vi "Create Frame Host LLP Packets.vi"(0 "frame configuration":T1={"pixel data type"=enum."RAW 8", "horizontal resolution"=0, "vertical resolution"=0, "virtual channel"=0.0, "include line sync packets"=FALSE}, 5 "frame number":u16, 11 "error in (no error)":errorcluster) -> (4 "frame packets":T3[](array[typedef]), 15 "error out":errorcluster)   [LabVIEW 2023, in "GettingStarted_Gen_148X_Host.lvlib"]
uses:
  GettingStarted_Gen_148X_Host.lvlib
  <instrlib>/FlexRIO/CSI-2/v2/Host/Types/Host LLP Packet.ctl
  <instrlib>/FlexRIO/CSI-2/v2/FPGA/Types/LLP Packet Header.ctl
  <instrlib>/FlexRIO/CSI-2/v2/FPGA/Types/LLP Packet Footer.ctl
  Types/Frame Data Configuration.ctl
  <instrlib>/FlexRIO/CSI-2/v2/Common/Types/LLP Data Type.ctl
  <instrlib>/FlexRIO/CSI-2/v2/FPGA/NI CSI-2 API FPGA v2.lvlib
  <instrlib>/FlexRIO/CSI-2/v2/Host/NI CSI-2 API Host v2.lvlib
  <instrlib>/FlexRIO/CSI-2/v2/Common/NI CSI-2 API Common v2.lvlib
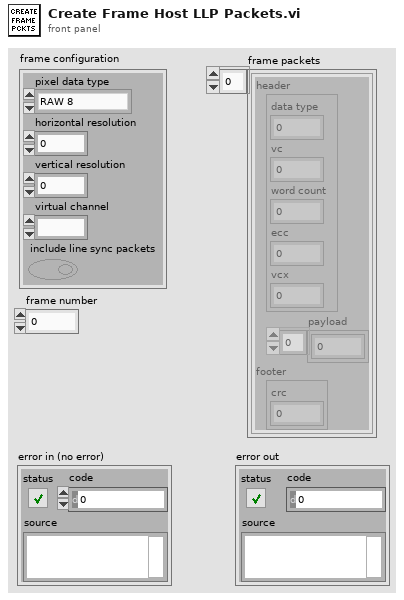
[diagram p1: front panel]
types:
  T1 = typedef "GettingStarted_Gen_148X_Host.lvlib/Frame Data Configuration.ctl" = cluster{"pixel data type":T2, "horizontal resolution":u16, "vertical resolution":u16, "virtual channel":fxp<+,4,4>, "include line sync packets":bool}
  T2 = typedef "NI CSI-2 API Common v2.lvlib/LLP Data Type.ctl" = enum8{"Frame Start", "Frame End", "Line Start", "Line End", "End of Transmission", "Reserved 0", "Reserved 1", "Reserved 2", "Generic Short Packet 1", "Generic Short Packet 2", "Generic Short Packet 3", "Generic Short Packet 4", "Generic Short Packet 5", "Generic Short Packet 6", "Generic Short Packet 7", "Generic Short Packet 8", "Null", "Blanking Data", "Embedded 8-bit non Image Data", "Generic Long Packet 1", "Generic Long Packet 2", "Generic Long Packet 3", "Generic Long Packet 4", "Reserved 3", "YUV420 8-bit", "YUV420 10-bit", "Legacy YUV420 8-bit", "Reserved 4", "YUV420 8-bit Chroma Shifted", "YUV420 10-bit Chroma Shifted", "YUV422 8-bit", "YUV422 10-bit", "RGB444", "RGB555", "RGB565", "RGB666", "RGB888", "Reserved 5", "Reserved 6", "RAW 24", "RAW 6", "RAW 7", "RAW 8", "RAW 10", "RAW 12", "RAW 14", "RAW 16", "RAW 20", "User Defined 8-bit Data 1", "User Defined 8-bit Data 2", "User Defined 8-bit Data 3", "User Defined 8-bit Data 4", "User Defined 8-bit Data 5", "User Defined 8-bit Data 6", "User Defined 8-bit Data 7", "User Defined 8-bit Data 8", "USL Command", "Reserved 7", "Reserved 8", "Reserved 9", "Reserved 10", "Reserved 11", "Reserved 12", "LRTE EPD Spacer"}
  T3 = typedef "NI CSI-2 API Host v2.lvlib/Host LLP Packet.ctl" = cluster{"header":T4, "payload":u8[], "footer":T5}
  T4 = typedef "NI CSI-2 API FPGA v2.lvlib/LLP Packet Header.ctl" = cluster{"word count":u16, "ecc":fxp<+,6,6>, "vcx":fxp<+,2,2>, "data type":fxp<+,6,6>, "vc":fxp<+,2,2>}
  T5 = typedef "NI CSI-2 API FPGA v2.lvlib/LLP Packet Footer.ctl" = cluster{"crc":u16}
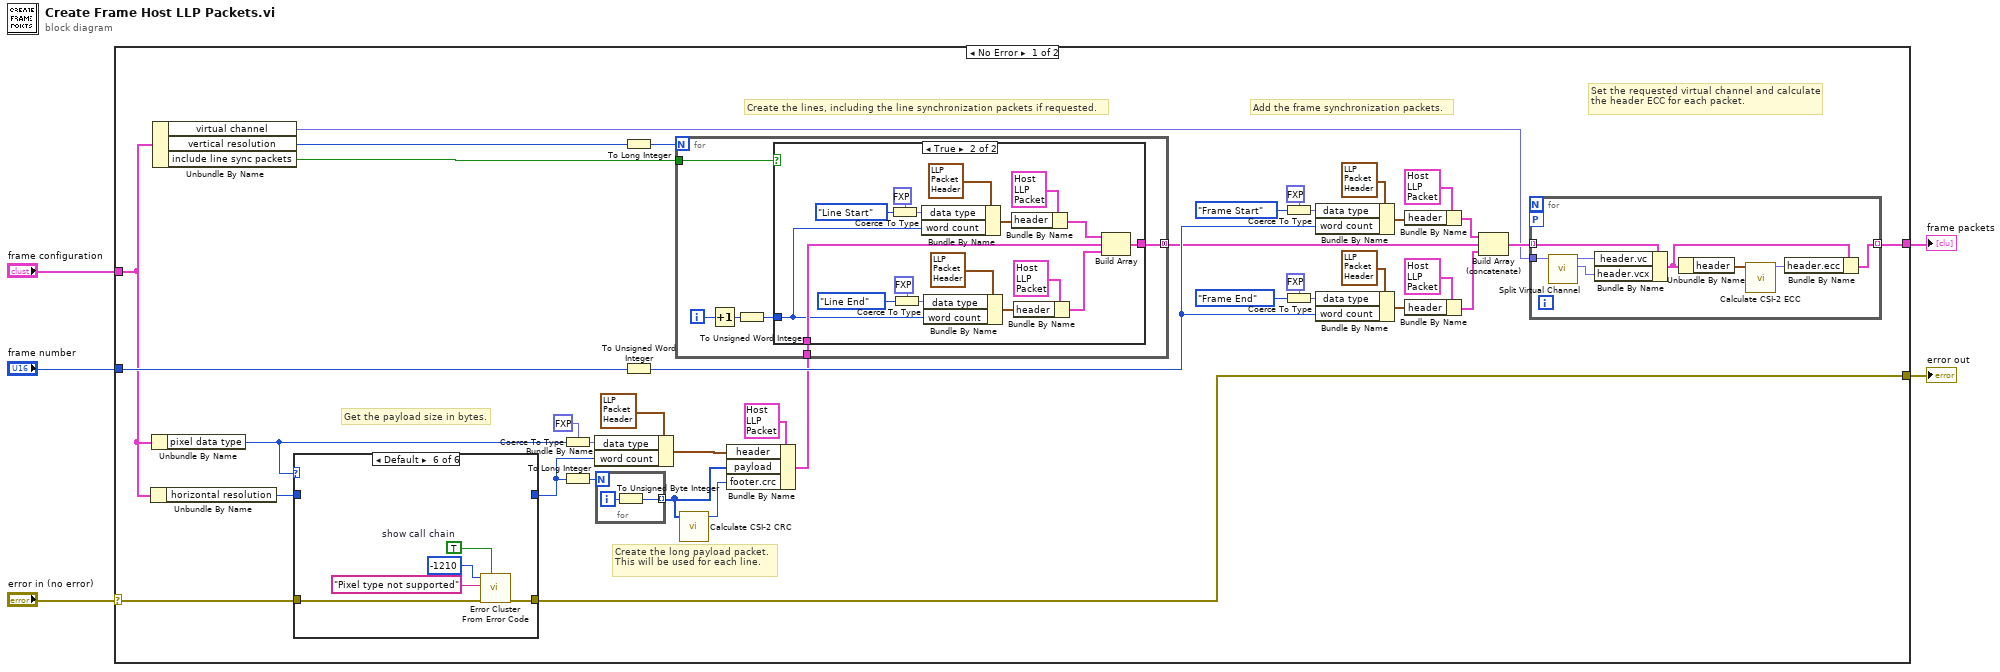
[diagram p0: block diagram]
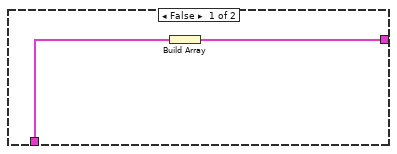
[diagram p2: hidden frame]
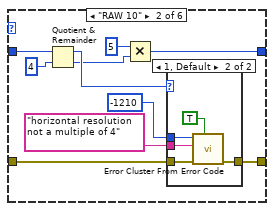
[diagram p4: hidden frame]
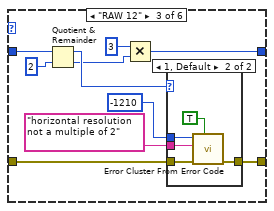
[diagram p6: hidden frame]
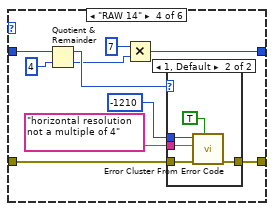
[diagram p8: hidden frame]
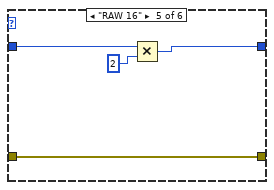
[diagram p10: hidden frame]
diagram:
  n1 = case shown="No Error" "error in (no error)" {
    selector: "error in (no error)" -> [w8 w138]
    tunnel: [w32 _] -> w5
    tunnel: [w43 w138] -> w3
    tunnel: "frame number" -> [w14 _]
    tunnel: "frame configuration" -> [w9 _]
    frame No Error {
      # "Set the requested virtual channel and calculate the header ECC for each packet."
      # "Add the frame synchronization packets."
      # "Create the lines, including the line synchronization packets if requested."
      # "Create the long payload packet.  This will be used for each line."
      # "Get the payload size in bytes."
      n2 = Unbundle By Name(w9) -> ("horizontal resolution"=w12:u16)
      n3 = Unbundle By Name(w9) -> ("pixel data type"=w13:T2)
      n4 = Unbundle By Name(w9) -> ("virtual channel"=w10:fxp<+,4,4>, "vertical resolution"=w11:u16, "include line sync packets"=w7:bool)
      n5 = case shown="Default" w13 {
        tunnel: w12 -> [w78 w81 w97 w113 w130 _]
        tunnel: [w78 w80 w96 w112 w128 _] -> w37
        tunnel: w8 -> [w77 w88 w104 w120 w127 w134]
        tunnel: [w77 w85 w101 w117 w127 w133] -> w43
        frame "RAW 8" {
        }
        frame "RAW 10" {
          n6 = Quotient & Remainder(x=w81, y=u16 4) -> (x-y*floor(x/y)=w83:u16, floor(x/y)=w79:u16)
          n7 = Multiply(x=u16 5 ("y"), y=w79) -> (x*y=w80:u16)
          n8 = case shown="1, Default" w83 {
            tunnel: w88 -> [w89 w91]
            tunnel: -1210 ("code") -> [_ w93]
            tunnel: "horizontal resolution not a multiple of 4" ("source") -> [_ w92]
            tunnel: [w89 w90] -> w85
            frame 0 {
            }
            frame 1, Default {
              n9 = call <vilib>:"Error Cluster From Error Code.vi"("show call chain? (False)"=TRUE ("show call chain"), "error in (no error)"=w91, "error message (\"\")"=w92, "error code (0)"=w93) -> ("error out"=w90:errorcluster)  [unwired: 5 in]
            }
          }
        }
        frame "RAW 12" {
          n10 = Quotient & Remainder(x=w97, y=u16 2) -> (x-y*floor(x/y)=w99:u16, floor(x/y)=w95:u16)
          n11 = Multiply(x=u16 3 ("y"), y=w95) -> (x*y=w96:u16)
          n12 = case shown="1, Default" w99 {
            tunnel: w104 -> [w105 w107]
            tunnel: -1210 ("code") -> [_ w109]
            tunnel: "horizontal resolution not a multiple of 2" ("source") -> [_ w108]
            tunnel: [w105 w106] -> w101
            frame 0 {
            }
            frame 1, Default {
              n13 = call <vilib>:"Error Cluster From Error Code.vi"("show call chain? (False)"=TRUE ("show call chain"), "error in (no error)"=w107, "error message (\"\")"=w108, "error code (0)"=w109) -> ("error out"=w106:errorcluster)  [unwired: 5 in]
            }
          }
        }
        frame "RAW 14" {
          n14 = Quotient & Remainder(x=w113, y=u16 4) -> (x-y*floor(x/y)=w115:u16, floor(x/y)=w111:u16)
          n15 = Multiply(x=u16 7 ("y"), y=w111) -> (x*y=w112:u16)
          n16 = case shown="1, Default" w115 {
            tunnel: w120 -> [w121 w123]
            tunnel: -1210 ("code") -> [_ w125]
            tunnel: "horizontal resolution not a multiple of 4" ("source") -> [_ w124]
            tunnel: [w121 w122] -> w117
            frame 0 {
            }
            frame 1, Default {
              n17 = call <vilib>:"Error Cluster From Error Code.vi"("show call chain? (False)"=TRUE ("show call chain"), "error in (no error)"=w123, "error message (\"\")"=w124, "error code (0)"=w125) -> ("error out"=w122:errorcluster)  [unwired: 5 in]
            }
          }
        }
        frame "RAW 16" {
          n18 = Multiply(x=w130, y=u16 2) -> (x*y=w128:u16)
        }
        frame Default {
          w135 = TRUE  # show call chain
          n19 = call <vilib>:"Error Cluster From Error Code.vi"("show call chain? (False)"=w135, "error in (no error)"=w134, "error message (\"\")"="Pixel type not supported" ("source"), "error code (0)"=-1210 ("code")) -> ("error out"=w133:errorcluster)  [unwired: 5 in]
        }
      }
      n20 = Coerce To Type(0:w13, 1:fxp<+,6,6> 0.0 ("data type")) -> (2:w40:fxp<+,6,6>)
      n21 = To Long Integer(number=w37) -> (32bit integer=w42:i32)
      n22 = Bundle By Name(cluster=T4 {"word count"=0, "ecc"=0.0, "vcx"=0.0, "data type"=0.0, "vc"=0.0} ("header"), "data type"=w40, "word count"=w37) -> (w41:T4)
      n23 = for {
        N: w42 -> [_]
        tunnel: [w136] -> w36 mode=indexing
        i -> [w137]
        n24 = To Unsigned Byte Integer(number=w137) -> (unsigned 8bit integer=w136:u8)
      }
      n25 = To Long Integer(number=w11) -> (32bit integer=w15:i32)
      n26 = To Unsigned Word Integer(number=w14) -> (unsigned 16bit integer=w19:u16)
      n27 = call <instrlib>:"Calculate CSI-2 CRC.vi"("payload"=w36) -> ("crc"=w35:u16)  [unwired: 10 in]
      n28 = Bundle By Name(cluster=T3 {"header"={"word count"=0, "ecc"=0.0, "vcx"=0.0, "data type"=0.0, "vc"=0.0}, "payload"=[], "footer"={"crc"=0}}, "header"=w41, "payload"=w36, "footer.crc"=w35) -> (w6:T3)
      n29 = for {
        N: w15 -> [_]
        tunnel: w7 -> [w45]
        tunnel: w6 -> [w46]
        tunnel: [w44] -> w18 mode=concatenating
        i -> [w47]
        n30 = Increment(x=w47) -> (x+1=w49:i32)
        n31 = To Unsigned Word Integer(number=w49) -> (unsigned 16bit integer=w48:u16)
        n32 = case shown="True" w45 {
          tunnel: w48 -> [_ w53]
          tunnel: w46 -> [w51 w55]
          tunnel: [w50 w52] -> w44
          frame False {
            n33 = Build Array(w51) -> (w50:T3[])
          }
          frame True {
            n34 = Coerce To Type(0:LLP_Data_Type."Line Start" ("Enum"), 1:fxp<+,6,6> 0.0 ("data type")) -> (2:w64:fxp<+,6,6>)
            n35 = Coerce To Type(0:LLP_Data_Type."Line End" ("Enum"), 1:fxp<+,6,6> 0.0 ("data type")) -> (2:w58:fxp<+,6,6>)
            n36 = Bundle By Name(cluster=T4 {"word count"=0, "ecc"=0.0, "vcx"=0.0, "data type"=0.0, "vc"=0.0} ("header"), "data type"=w64, "word count"=w53) -> (w67:T4)
            n37 = Bundle By Name(cluster=T4 {"word count"=0, "ecc"=0.0, "vcx"=0.0, "data type"=0.0, "vc"=0.0} ("header"), "data type"=w58, "word count"=w53) -> (w61:T4)
            n38 = Bundle By Name(cluster=T3 {"header"={"word count"=0, "ecc"=0.0, "vcx"=0.0, "data type"=0.0, "vc"=0.0}, "payload"=[], "footer"={"crc"=0}}, "header"=w67) -> (w56:T3)
            n39 = Bundle By Name(cluster=T3 {"header"={"word count"=0, "ecc"=0.0, "vcx"=0.0, "data type"=0.0, "vc"=0.0}, "payload"=[], "footer"={"crc"=0}}, "header"=w61) -> (w54:T3)
            n40 = Build Array(w56, w55, w54) -> (w52:T3[])
          }
        }
      }
      n41 = Coerce To Type(0:LLP_Data_Type."Frame Start" ("Enum"), 1:fxp<+,6,6> 0.0 ("data type")) -> (2:w25:fxp<+,6,6>)
      n42 = Coerce To Type(0:LLP_Data_Type."Frame End" ("Enum"), 1:fxp<+,6,6> 0.0 ("data type")) -> (2:w26:fxp<+,6,6>)
      n43 = Bundle By Name(cluster=T4 {"word count"=0, "ecc"=0.0, "vcx"=0.0, "data type"=0.0, "vc"=0.0} ("header"), "data type"=w25, "word count"=w19) -> (w22:T4)
      n44 = Bundle By Name(cluster=T4 {"word count"=0, "ecc"=0.0, "vcx"=0.0, "data type"=0.0, "vc"=0.0} ("header"), "data type"=w26, "word count"=w19) -> (w29:T4)
      n45 = Bundle By Name(cluster=T3 {"header"={"word count"=0, "ecc"=0.0, "vcx"=0.0, "data type"=0.0, "vc"=0.0}, "payload"=[], "footer"={"crc"=0}}, "header"=w22) -> (w17:T3)
      n46 = Bundle By Name(cluster=T3 {"header"={"word count"=0, "ecc"=0.0, "vcx"=0.0, "data type"=0.0, "vc"=0.0}, "payload"=[], "footer"={"crc"=0}}, "header"=w29) -> (w16:T3)
      n47 = Build Array (concatenate)(w17, w18, w16) -> (w33:T3[])
      n48 = for {
        tunnel: w33 -> [w76] mode=indexing
        tunnel: w10 -> [w73]
        tunnel: [w69] -> w32 mode=indexing
        workers-P: _ -> [_]
        n49 = call <instrlib>:"Split Virtual Channel.vi"("virtual channel"=w73) -> ("vcx"=w74:fxp<+,2,2>, "vc"=w75:fxp<+,2,2>)  [unwired: 9 in]
        n50 = Bundle By Name(cluster=w76, "header.vc"=w75, "header.vcx"=w74) -> (w70:T3)
        n51 = Unbundle By Name(w70) -> ("header"=w72:T4)
        n52 = call <instrlib>:"Calculate CSI-2 ECC.vi"("header"=w72) -> ("ecc"=w71:fxp<+,6,6>)  [unwired: 10 in]
        n53 = Bundle By Name(cluster=w70, "header.ecc"=w71) -> (w69:T3)
      }
    }
    frame Error {
    }
  }
  "error out" <- w3
  "frame packets" <- w5
